vi "Read Alarm Limits are Active.vi"(8 "error in":errorcluster, 11 "Has Alarm Limits in":refnum<class "Has Alarm Limits.lvclass">) -> (0 "error out":errorcluster, 2 "alarm limits active?":bool, 3 "Has Alarm Limits out":refnum<class "Has Alarm Limits.lvclass">)   [LabVIEW 2020, in "PV Access.lvlib" / "PV Data.lvlib" / "Has Alarm Limits.lvclass"]
uses:
  Has Alarm Limits.lvclass
  182da66a-f6ee-47d3-9b05-9cecdf4c7a27.vi
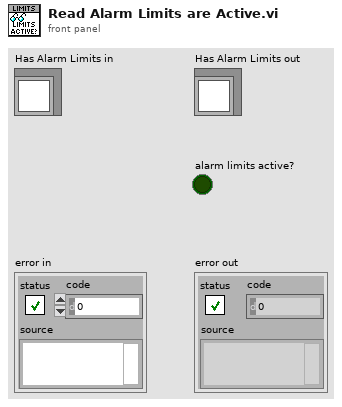
[diagram p1: front panel]
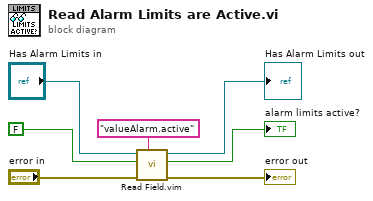
[diagram p0: block diagram]
diagram:
  n1 = call "Read Field.vim"("field"="valueAlarm.active" ("element name"), "error in"="error in", "default value"=FALSE, "Base Interface in"="Has Alarm Limits in") -> ("error out"=→"error out":errorcluster, "value"=→"alarm limits active?":bool, "Base Interface out"=→"Has Alarm Limits out":refnum<class "Has Alarm Limits.lvclass">)  [unwired: 5 in]
